vi "Page_Source_Add_Update_Dest_and_Inclusion.vi"(6 "send to main destination?":bool, 8 "error in (no error)":errorcluster, 10 "Inclusion":T1, 11 "AB_Source_VI in":refnum<class "AB_Source.lvclass">) -> (0 "error out":errorcluster, 1 "itemID":string, 3 "AB_Source_VI out":refnum<class "AB_Source.lvclass">)   [LabVIEW 2020, in "AB_Source.lvclass"]
uses:
  <vilib>/AppBuilder/AB_Classes/Source/AB_Source.lvclass
  <vilib>/AppBuilder/AB_Source_Inclusion.ctl
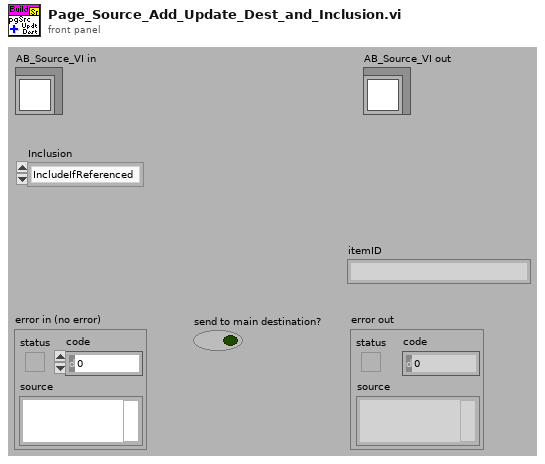
[diagram p1: front panel]
types:
  T1 = typedef "AB_Source_Inclusion.ctl" = enum16{"IncludeIfReferenced", "Include", "Exclude", "TopLevel"}
  T2 = typedef "AB_Source.ctl" = cluster{"path":path, "itemID":string, "parentIndex":i32, "sourceInclusion":T1, "destinationIndex":i32, "properties":T3[], "newName":string, "lvfile":bool, "valid":bool, "eng_inBuild":bool, "eng_isNonVILink":bool, "Amalgamation":bool, "Amalgamation Piece":bool, "eng_delimitedName":string, "preventRename":bool}
  T3 = typedef "AB_Source_Properties.ctl" = cluster{"sourcePropertyType":T4, "value":variant}
  T4 = typedef "AB_Source_Property_Type.ctl" = enum16{"Remove block diagram", "Remove front panel", "Password", "Window has title bar", "Show menu bar", "Show vertical scroll bar", "Show horizontal scroll bar", "Show toolbar", "Show Abort button", "Show fp when called", "Window behavior", "Allow user to close window", "Window run-time position", "Run when opened", "Allow debugging", "Auto error handling", "Generate guard code", "Use stack variables", "Expression folding", "Integer only", "Inline subVI"}
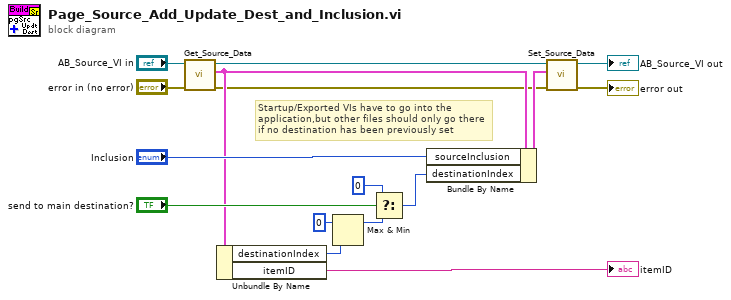
[diagram p0: block diagram]
diagram:
  # "Startup/Exported VIs have to go into the application,but other files should only go there if no destination has been previously set"
  n1 = call <vilib>:"Get_Source_Data.vi"("error in (no error)"="error in (no error)", "Class in"="AB_Source_VI in") -> ("error out"=w2:errorcluster, "data"=w4:T2, "Class out"=w6:refnum<class "AB_Source.lvclass">)  [unwired: 7 in]
  n2 = Unbundle By Name(w4) -> ("destinationIndex"=w13:i32, "itemID"=→"itemID":string)
  n3 = Max & Min(x=0 ("destinationIndex"), y=w13) -> (max(x,y)=w14:i32)  [unwired: 1 out]
  n4 = Select(t=0 ("destinationIndex"), s="send to main destination?", f=w14) -> (s? t:f=w16:i32)
  n5 = Bundle By Name(cluster=w4, "sourceInclusion"="Inclusion", "destinationIndex"=w16) -> (w5:T2)
  n6 = call <vilib>:"Set_Source_Data.vi"("error in (no error)"=w2, "data"=w5, "Class in"=w6) -> ("error out"=→"error out":errorcluster, "Class out"=→"AB_Source_VI out":refnum<class "AB_Source.lvclass">)  [unwired: 7 in]
